vi "Advance Query Adjust In built table.vi"(8 "error in (no error)":errorcluster, 10 "Database in":refnum<class "Database.lvclass">, 11 "UserInfoManageUI":refnum<class "UserInfoManageUI.lvclass">) -> (0 "error out":errorcluster, 3 "UserInfoManageUI out":refnum<class "UserInfoManageUI.lvclass">)   [LabVIEW 2015, in "ActorManagement.lvlib" / "UserInfoManageUI.lvclass"]
uses:
  UserInfoManageUI.lvclass
  DatabaseManagement/Database.lvclass
  PluginWithDatabase/PluginWithDatabase.lvclass/PluginWithDatabase.ctl
  UserManagement/Model/Model.lvclass
  PluginWithDatabase/PluginWithDatabase.lvclass
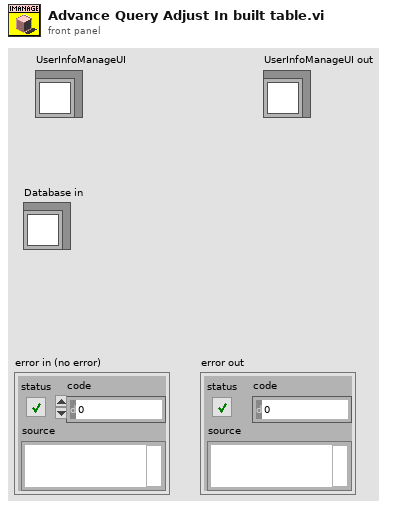
[diagram p1: front panel]
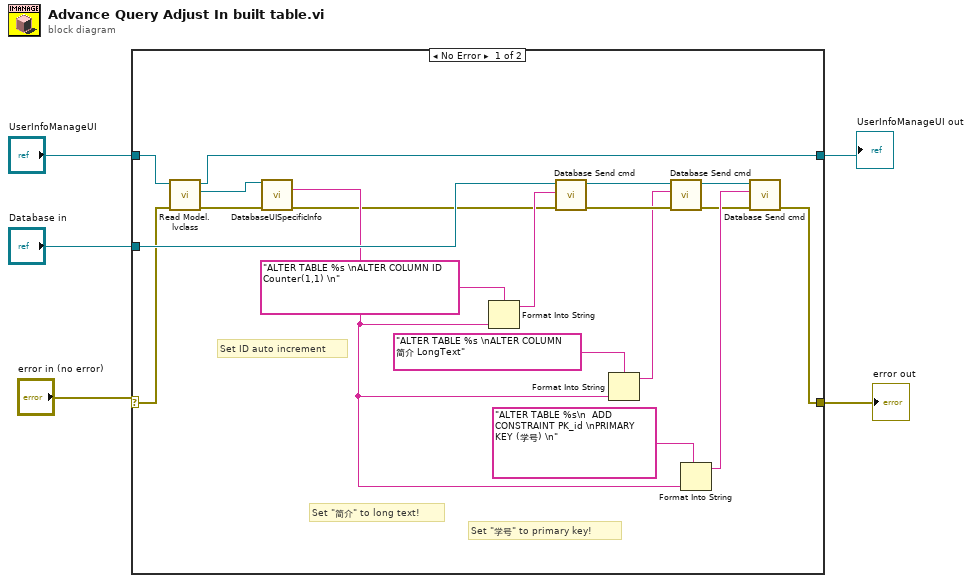
[diagram p0: block diagram]
diagram:
  n1 = case shown="No Error" "error in (no error)" {
    selector: "error in (no error)" -> [w11 w26]
    tunnel: [w24 w26] -> w1
    tunnel: "UserInfoManageUI" -> [w12 w25]
    tunnel: "Database in" -> [w14 _]
    tunnel: [w6 w25] -> w2
    frame No Error {
      # "Set \"学号\" to primary key!"
      # "Set \"简介\" to long text!"
      # "Set ID auto increment"
      n2 = call "Read Model.lvclass.vi"("error in (no error)"=w11, "PluginWithDatabase in"=w12) -> ("error out"=w7:errorcluster, "UserManagement.lvlib:Model"=w10:refnum<class "Model.lvclass">, "PluginWithDatabase out"=w6:refnum<class "UserInfoManageUI.lvclass">)  [unwired: 7 in]
      n3 = call-dynamic "DatabaseUISpecificInfo.vi"("Model.lvclass"=w10, "error in (no error)"=w7) -> ("TableName"=w9:string, "error out"=w8:errorcluster)  [unwired: 9 in, 3 out]
      n4 = Format Into String(format string="ALTER TABLE %s \nALTER COLUMN ID Counter(1,1) \n" ("SQL query"), w9) -> (resulting string=w20:string)  [unwired: 2 in, 1 out]
      n5 = call "Database Send cmd.vi"("error in (no error)"=w8, "SQL query"=w20, "Database in"=w14) -> ("error out"=w17:errorcluster, "Database out"=w18:refnum<class "Database.lvclass">)  [unwired: 7 in]
      n6 = Format Into String(format string="ALTER TABLE %s \nALTER COLUMN 简介 LongText" ("SQL query"), w9) -> (resulting string=w13:string)  [unwired: 2 in, 1 out]
      n7 = call "Database Send cmd.vi"("error in (no error)"=w17, "SQL query"=w13, "Database in"=w18) -> ("error out"=w15:errorcluster, "Database out"=w16:refnum<class "Database.lvclass">)  [unwired: 7 in]
      n8 = Format Into String(format string="ALTER TABLE %s\n  ADD CONSTRAINT PK_id \nPRIMARY KEY (学号) \n" ("SQL query"), w9) -> (resulting string=w19:string)  [unwired: 2 in, 1 out]
      n9 = call "Database Send cmd.vi"("error in (no error)"=w15, "SQL query"=w19, "Database in"=w16) -> ("error out"=w24:errorcluster)  [unwired: 7 in, 1 out]
    }
    frame Error {
    }
  }
  "error out" <- w1
  "UserInfoManageUI out" <- w2
